vi "SetChanged.vi"(9 "changed?":bool, 10 "VI Index":i32, 11 "Array in":T1[](array[typedef])) -> (3 "Array out":T1[](array[typedef]))   [LabVIEW 2016, in "update vi properties.lvlib"]
uses:
  update vi properties.lvlib
  Cluster_Data.ctl
  <vilib>/picture/picture.llb/imagedata.ctl
panel:
  # "Connector Pane"
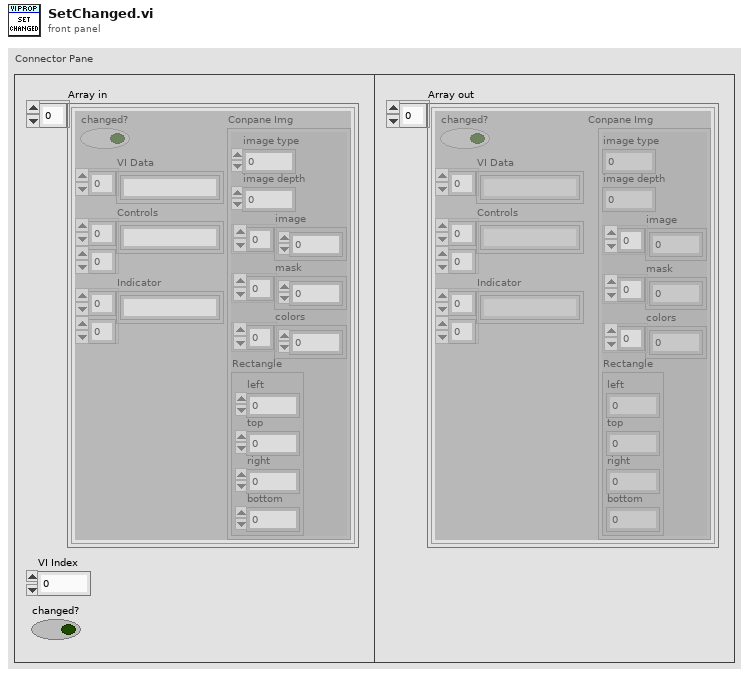
[diagram p1: front panel]
types:
  T1 = typedef "update vi properties.lvlib/Cluster_Data.ctl" = cluster{"changed?":bool, "VI Data":string[], "Controls":string[][], "Indicator":string[][], "Conpane Img":T2}
  T2 = typedef "imagedata.ctl" = cluster{"image type":i32, "image depth":i32, "image":u8[], "mask":u8[], "colors":u32[], "Rectangle":cluster{"left":i16, "top":i16, "right":i16, "bottom":i16}}
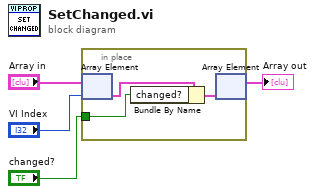
[diagram p0: block diagram]
diagram:
  n1 = in-place {
    in-place-border: "changed?" -> [w5]
    n2 = in-place-array #1("Array in", "VI Index") -> (w7:T1)
    n3 = Bundle By Name(cluster=w7, "changed?"=w5) -> (w6:T1)
    n4 = in-place-array #1(w6) -> (→"Array out":T1[])  [unwired: 1 out]
  }
